vi "TimeInPast.vi"() -> (0 "Time Stamp":timestamp)   [LabVIEW 2015, in "Exposure Process.lvlib"]
uses:
  Exposure Process.lvlib
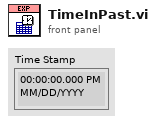
[diagram p1: front panel]
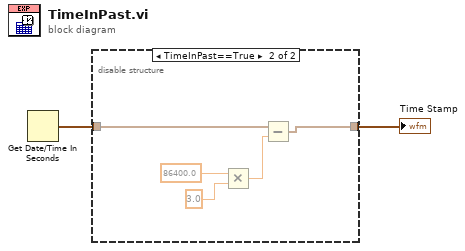
[diagram p0: block diagram]
diagram:
  n1 = Get Date/Time In Seconds() -> (seconds since 1Jan1904=w2:timestamp)
  n2 = disable-structure shown="TimeInPast==True" {
    disable-tunnel: w2 -> [w3 w7]
    disable-tunnel: [w3 w4] -> w1
    frame condition #0 (active) {
    }
    frame condition #1 {
      n3 = Multiply(x=86400.0, y=3.0) -> (x*y=w6:dbl)
      n4 = Subtract(x=w7, y=w6) -> (x-y=w4:timestamp)
    }
  }
  "Time Stamp" <- w1
